vi "Fecha_HMI.vi"() -> (3 "fecha y hora":T1)   [LabVIEW 2018]
uses:
  Controls/Hora y Fecha control.ctl
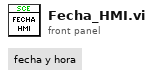
[diagram p1: front panel]
types:
  T1 = typedef "Hora y Fecha control.ctl" = cluster{"fecha":string, "dia semana":string, "fecha 2":string}
  T2 = cluster{"date/time string":string, "date/time string":string, string}
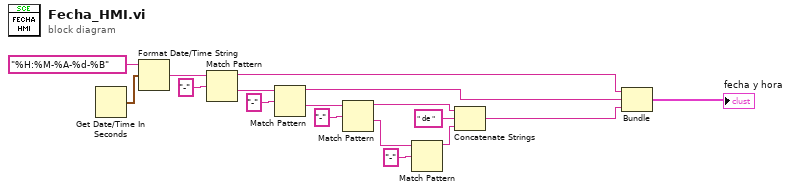
[diagram p0: block diagram]
diagram:
  n1 = Get Date/Time In Seconds() -> (seconds since 1Jan1904=w16:timestamp)
  n2 = Format Date/Time String(time format string (%c)="%H:%M-%A-%d-%B", seconds (now)=w16) -> (date/time string=w15:string)  [unwired: 1 in]
  n3 = Match Pattern(string=w15, regular expression="-") -> (before substring=w4:string, after substring=w12:string)  [unwired: 1 in, 2 out]
  n4 = Match Pattern(string=w12, regular expression="-") -> (before substring=w3:string, after substring=w10:string)  [unwired: 1 in, 2 out]
  n5 = Match Pattern(string=w10, regular expression="-") -> (before substring=w7:string, after substring=w8:string)  [unwired: 1 in, 2 out]
  n6 = Match Pattern(string=w8, regular expression="-") -> (before substring=w5:string)  [unwired: 1 in, 3 out]
  n7 = Concatenate Strings(w7, " de " ("string"), w5) -> (w2:string)
  n8 = Bundle("date/time string"=w4, "date/time string"=w3, w2) -> (→"fecha y hora":T2)  [unwired: 1 in]
